vi "ProductionStatusInit.vi"() -> (1 "DataSource Data":string[][](table), 2 "ColumnSetup":T1[](array[typedef]) {"MinWidth" min=2 step=1; "AutoSizeMode" items=["None"=1, "ColumnHeader"=2, "AllCellsExceptHeader"=4, "AllCells"=6, "DisplayedCellsExceptHeader"=8, "DisplayedCells"=10, "Fill"=16]; "FillWeight" min=1 max=100})   [LabVIEW 2020]
uses:
  <vilib>/DataGrid for LabVIEW/source/GridColumn/ColumnDefinition.ctl
  <vilib>/DataGrid for LabVIEW/source/GridColumn/ColumnType.ctl
  <vilib>/DataGrid for LabVIEW/source/GridColumn/GridColumn.lvclass
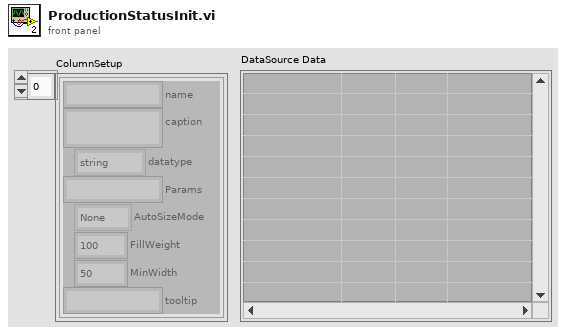
[diagram p1: front panel]
types:
  T1 = typedef "DataGrid.lvlib/GridColumn.lvclass/ColumnDefinition.ctl" = cluster{"name":string, "caption":string, "datatype":T2, "Params":string, "AutoSizeMode":i32, "FillWeight":sgl, "MinWidth":u32, "tooltip":string}
  T2 = typedef "DataGrid.lvlib/GridColumn.lvclass/ColumnType.ctl" = enum16{"string", "image", "check", "numeric", "timestamp", "button", "combo", "link"}
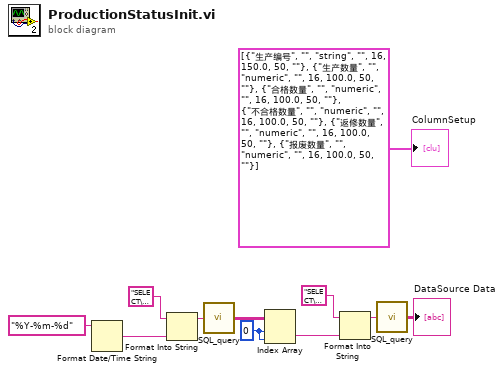
[diagram p0: block diagram]
diagram:
  w4 = 0 ("索引 (行)")
  n1 = Format Date/Time String(time format string (%c)="%Y-%m-%d" ("时间格式字符串(%c)")) -> (date/time string=w7:string)  [unwired: 2 in]
  n2 = Format Into String(format string="SELECT\ndbo.[生产计划].[生产编号]\n\nFROM\ndbo.[生产计划]\nWHERE\ndbo.[生产计划].[日期] = N'%s'\n", w7) -> (resulting string=w6:string)  [unwired: 2 in, 1 out]
  n3 = call "SQL_query.vi"("SQL query"=w6) -> ("data"=w5:string[][])  [unwired: 3 in, 1 out]
  n4 = Index Array(array=w5, index (row)=w4, index (col)=w4) -> (element=w2:string)
  n5 = Format Into String(format string="SELECT\ndbo.[产量].[生产编号],\ndbo.[产量].[生产数量],\ndbo.[产量].[合格数量],\ndbo.[产量].[不合格数量],\ndbo.[产量].[返修数量],\ndbo.[产量].[报废数量]\n\nFROM\ndbo.[产量]\nWHERE\ndbo.[产量].[生产编号] = N'%s'\n" ("SQL query"), w2) -> (resulting string=w1:string)  [unwired: 2 in, 1 out]
  n6 = call "SQL_query.vi"("SQL query"=w1) -> ("data"=→"DataSource Data":string[][])  [unwired: 3 in, 1 out]
  "ColumnSetup" <- T1[] [{"name"="生产编号", "caption"="", "datatype"=enum."string", "Params"="", "AutoSizeMode"=16, "FillWeight"=150.0, "MinWidth"=50, "tooltip"=""}, {"name"="生产数量", "caption"="", "datatype"=enum."numeric", "Params"="", "AutoSizeMode"=16, "FillWeight"=100.0, "MinWidth"=50, "tooltip"=""}, {"name"="合格数量", "caption"="", "datatype"=enum."numeric", "Params"="", "AutoSizeMode"=16, "FillWeight"=100.0, "MinWidth"=50, "tooltip"=""}, {"name"="不合格数量", "caption"="", "datatype"=enum."numeric", "Params"="", "AutoSizeMode"=16, "FillWeight"=100.0, "MinWidth"=50, "tooltip"=""}, {"name"="返修数量", "caption"="", "datatype"=enum."numeric", "Params"="", "AutoSizeMode"=16, "FillWeight"=100.0, "MinWidth"=50, "tooltip"=""}, {"name"="报废数量", "caption"="", "datatype"=enum."numeric", "Params"="", "AutoSizeMode"=16, "FillWeight"=100.0, "MinWidth"=50, "tooltip"=""}] ("ColumnSetup")
